vi "Write Button.vi"(6 "Button":u16, 11 "Handle Mouse Down Msg in":refnum<class "Handle Mouse Down Msg.lvclass">) -> (3 "Handle Mouse Down Msg out":refnum<class "Handle Mouse Down Msg.lvclass">)   [LabVIEW 2017, in "Handle Mouse Down Msg.lvclass"]
uses:
  <vilib>/gpm_packages/@cs/Test-executive-builder/Source/Test Executive Builder View/Test Executive Builder View Messages/Handle Mouse Down Msg/Handle Mouse Down Msg.lvclass
  <vilib>/gpm_packages/@cs/Test-executive-builder/Source/Test Executive Builder View/Test Executive Builder View Messages/Handle Mouse Down Msg/Handle Mouse Down Msg.lvclass/Handle Mouse Down Msg.ctl
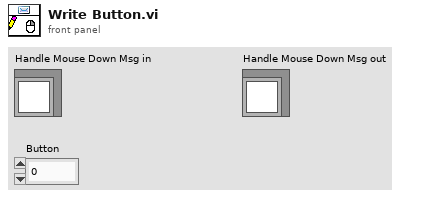
[diagram p1: front panel]
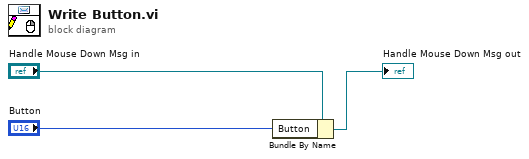
[diagram p0: block diagram]
diagram:
  n1 = Bundle By Name(cluster="Handle Mouse Down Msg in", "Button"="Button") -> (→"Handle Mouse Down Msg out":refnum<class "Handle Mouse Down Msg.lvclass">)
